vi "Display Information.vi"(8 "error in (no error)":errorcluster, 10 "Select Recipe":u16(ring) items=["1234567hjed", "tswri", "ad975t", "6yt"], 11 "Master in":refnum<class "Master.lvclass">) -> (0 "error out":errorcluster, 1 "Total Yields":dbl, 2 "Recipe":T2(array[cluster]), 3 "Master out":refnum<class "Master.lvclass">, 5 "Parameter":T1, 6 "Production Record":T3(array[cluster]))   [LabVIEW 2014, in "Master.lvclass"]
uses:
  Master/Master.lvclass
  Master/Master.lvclass/Master.ctl
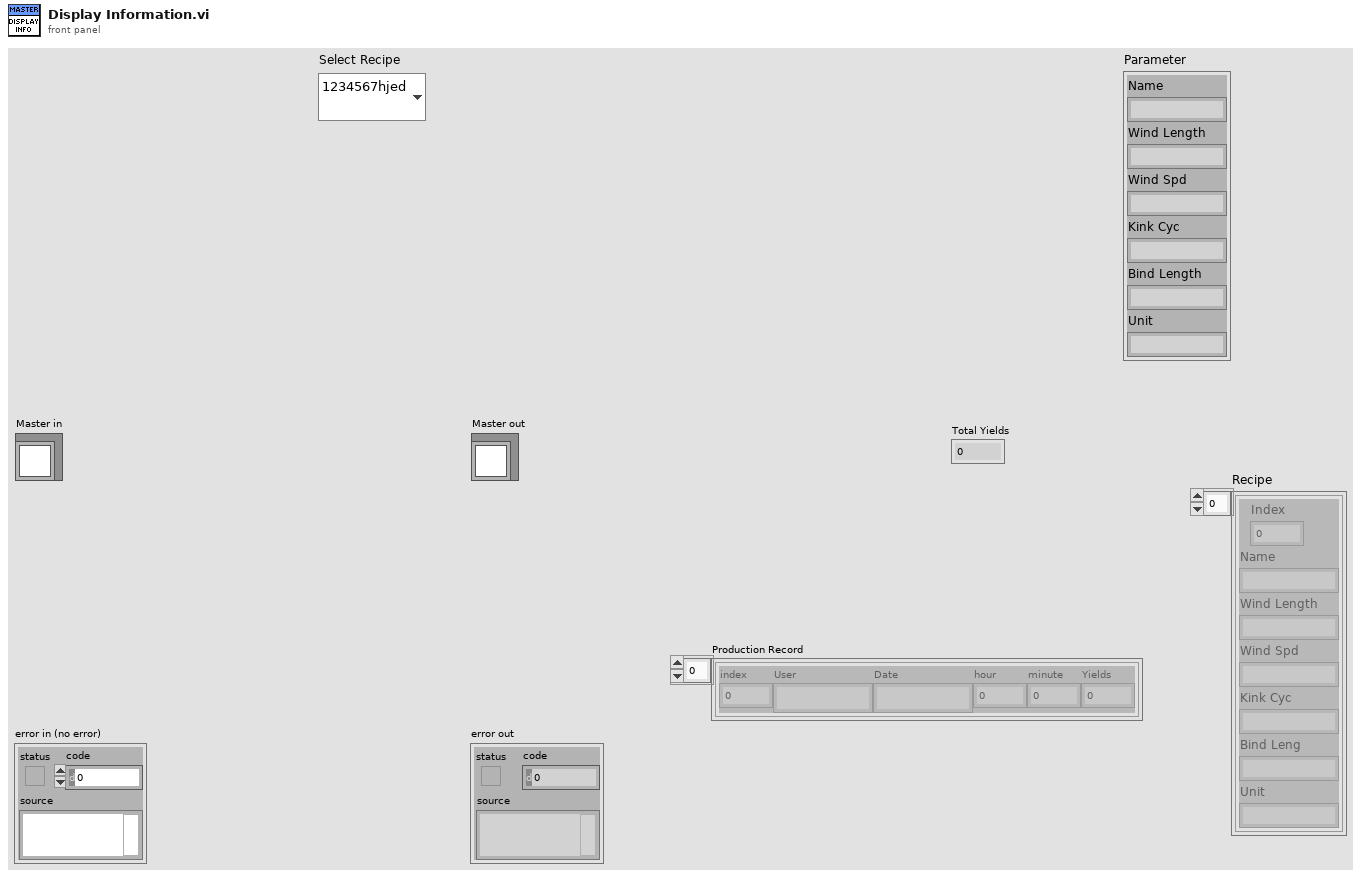
[diagram p1: front panel]
types:
  T1 = cluster{"Name":string, "Wind Length":string, "Wind Spd":string, "Kink Cyc":string, "Bind Length":string, "Unit":string}
  T2 = cluster{"Index":i32, "Name":string, "Wind Length":string, "Wind Spd":string, "Kink Cyc":string, "Bind Leng":string, "Unit":string}[]
  T3 = cluster{"index":i32, "User":string, "Date":string, "hour":i32, "minute":i32, "Yields":dbl}[]
  T4 = cluster{"User":string, "Date":string, "Yields":dbl, "hour":i32, "minute":i32}[]
  T5 = cluster{"Name":string, "Wind Length":string, "Wind Spd":string, "Kink Cyc":string, "Bind Length":string, "Unit":string}[]
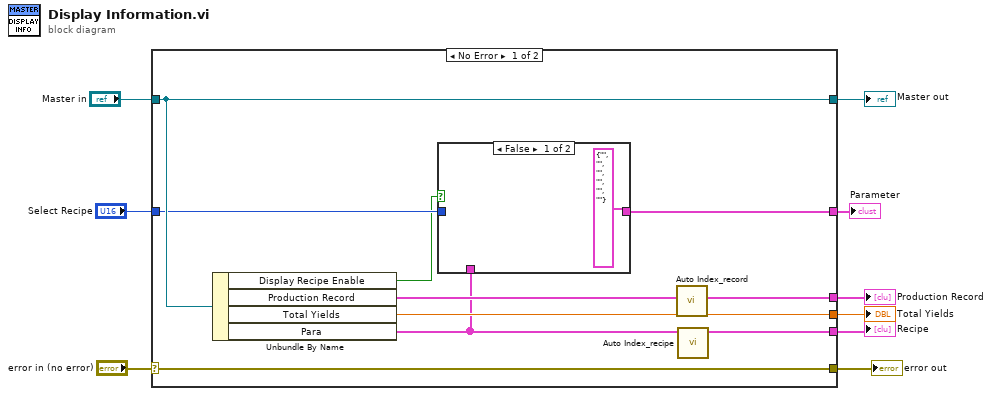
[diagram p0: block diagram]
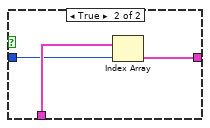
[diagram p2: hidden frame]
diagram:
  n1 = case shown="No Error" "error in (no error)" {
    selector: "error in (no error)" -> [w19 w24]
    tunnel: [w19 w24] -> w8
    tunnel: [w16 w25] -> w6
    tunnel: "Master in" -> [w16 w25]
    tunnel: [w17 _] -> w5
    tunnel: [w18 _] -> w4
    tunnel: [w15 _] -> w3
    tunnel: "Select Recipe" -> [w12 _]
    tunnel: [w10 _] -> w1
    frame No Error {
      n2 = Unbundle By Name(w16) -> ("Display Recipe Enable"=w11:bool, "Production Record"=w14:T4, "Total Yields"=w18:dbl, "Para"=w13:T5)
      n3 = case shown="False" w11 {
        tunnel: w13 -> [_ w23]
        tunnel: w12 -> [_ w22]
        tunnel: [T1 {"Name"="", "Wind Length"="", "Wind Spd"="", "Kink Cyc"="", "Bind Length"="", "Unit"=""} ("Parameter") w21] -> w10
        frame False {
        }
        frame True {
          n4 = Index Array(array=w23, index=w22) -> (element=w21:T1)
        }
      }
      n5 = call "Auto Index_record.vi"("User                   Date                 hr     min      Yields"=w14) -> ("Array"=w17:T3)  [unwired: 10 in]
      n6 = call "Auto Index_recipe.vi"("New Recipe.Para"=w13) -> ("Array"=w15:T2)  [unwired: 10 in]
    }
    frame Error {
    }
  }
  "error out" <- w8
  "Master out" <- w6
  "Total Yields" <- w4
  "Production Record" <- w5
  "Recipe" <- w3
  "Parameter" <- w1
